vi "Get Status.vi"(9 "Error message input":string, 10 "Input Pump Status string":string, 11 "Input Status String":string) -> (1 "Error message string":string, 2 "Output Pump Status":string, 3 "Output Status String":string)   [LabVIEW 2013]
panel:
  out "Error Status":bool[](array[boolean])
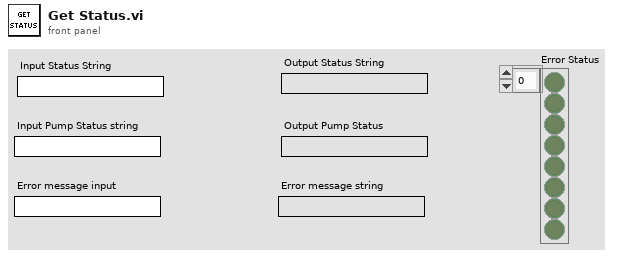
[diagram p1: front panel]
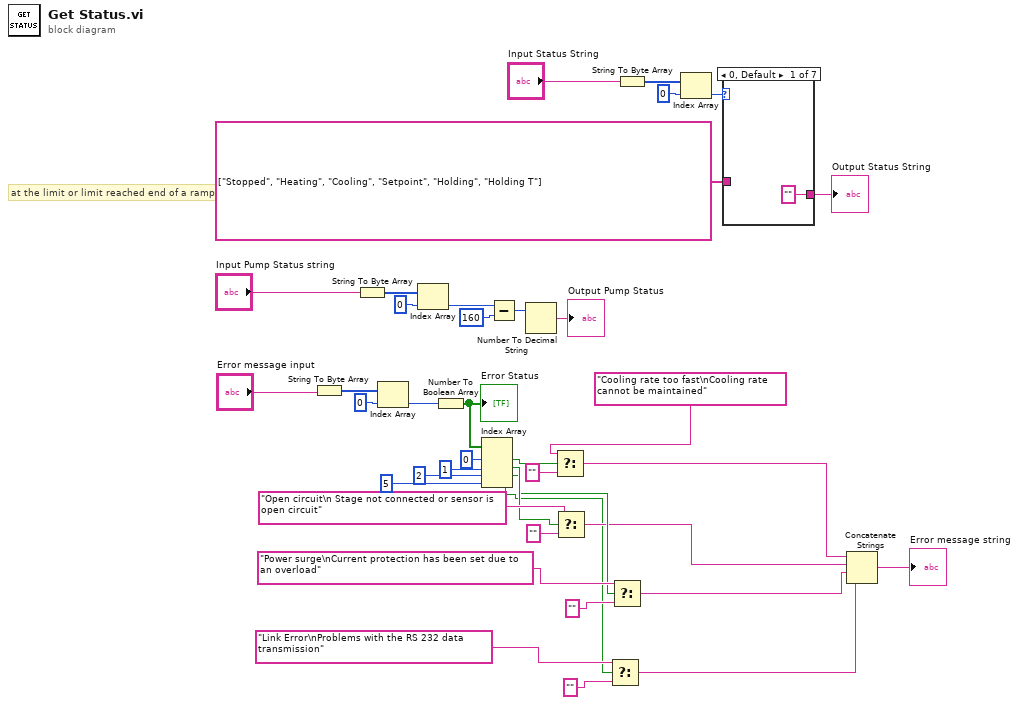
[diagram p0: block diagram]
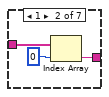
[diagram p2: hidden frame]
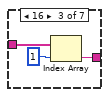
[diagram p3: hidden frame]
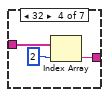
[diagram p4: hidden frame]
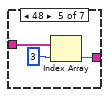
[diagram p5: hidden frame]
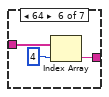
[diagram p6: hidden frame]
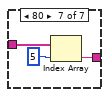
[diagram p7: hidden frame]
diagram:
  # "at the limit or limit reached end of a ramp"
  n1 = String To Byte Array(string="Error message input") -> (unsigned byte array=w25:u8[])
  n2 = String To Byte Array(string="Input Pump Status string") -> (unsigned byte array=w32:u8[])
  n3 = Index Array(array=w25, index=0) -> (element=w23:u8)
  n4 = Index Array(array=w32, index=0) -> (element=w30:u8)
  n5 = Number To Boolean Array(number=w23) -> (Boolean array=w22:bool[])
  "Error Status" <- w22
  n6 = Index Array(array=w22, index #1=0 ("index"), index #2=1 ("index"), index #3=2 ("index"), index #4=5 ("index")) -> (element #1=w17:bool, element #2=w11:bool, element #3=w10:bool, element #4=w1:bool)
  n7 = Subtract(x=w30, y=u8 160) -> (x-y=w28:u8)
  n8 = Number To Decimal String(number=w28) -> (decimal integer string=→"Output Pump Status":string)  [unwired: 1 in]
  n9 = Select(t="Cooling rate too fast\nCooling rate cannot be maintained", s=w17, f="") -> (s? t:f=w8:string)
  n10 = Select(t="Open circuit\n Stage not connected or sensor is open circuit", s=w11, f="") -> (s? t:f=w7:string)
  n11 = Select(t="Link Error\nProblems with the RS 232 data transmission", s=w1, f="") -> (s? t:f=w3:string)
  n12 = Select(t="Power surge\nCurrent protection has been set due to an overload", s=w10, f="") -> (s? t:f=w6:string)
  n13 = String To Byte Array(string="Input Status String") -> (unsigned byte array=w39:u8[])
  n14 = Index Array(array=w39, index=0) -> (element=w36:u8)
  n15 = case shown="0, Default" w36 {
    tunnel: string[] ["Stopped", "Heating", "Cooling", "Setpoint", "Holding", "Holding T"] -> [_ w43 w46 w49 w52 w55 w58]
    tunnel: ["" w41 w44 w47 w50 w53 w56] -> w34
    frame 0, Default {
    }
    frame 1 {
      n16 = Index Array(array=w43, index=0) -> (element=w41:string)
    }
    frame 16 {
      n17 = Index Array(array=w46, index=1) -> (element=w44:string)
    }
    frame 32 {
      n18 = Index Array(array=w49, index=2) -> (element=w47:string)
    }
    frame 48 {
      n19 = Index Array(array=w52, index=3) -> (element=w50:string)
    }
    frame 64 {
      n20 = Index Array(array=w55, index=4) -> (element=w53:string)
    }
    frame 80 {
      n21 = Index Array(array=w58, index=5) -> (element=w56:string)
    }
  }
  "Output Status String" <- w34
  n22 = Concatenate Strings(w8, w7, w6, w3) -> (→"Error message string":string)
